vi "Initialize.vi"(8 "error in (no error)":errorcluster, 11 "Simple Actor in":refnum<class "Simple Actor.lvclass">) -> (0 "error out":errorcluster, 3 "Simple Actor out":refnum<class "Simple Actor.lvclass">)   [LabVIEW 2020, in "Simple Actor.lvlib" / "Simple Actor.lvclass"]
uses:
  Simple Actor.lvclass
  Execute Msg/Execute Msg.lvclass
  E:/NI I Program/Actor Intr Demo/Simple Actor/Actor Msg/Actor Msg.lvclass
  Simple Actor.lvclass/Simple Actor.ctl
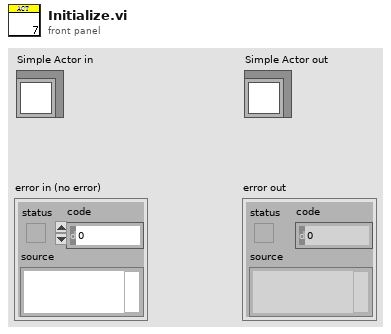
[diagram p1: front panel]
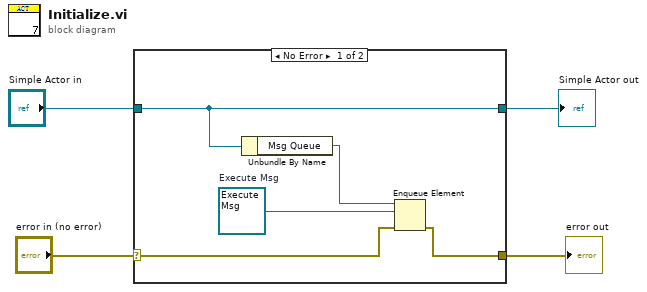
[diagram p0: block diagram]
diagram:
  n1 = case shown="No Error" "error in (no error)" {
    selector: "error in (no error)" -> [w6 w11]
    tunnel: [w5 w11] -> w3
    tunnel: [w9 w10] -> w1
    tunnel: "Simple Actor in" -> [w9 w10]
    frame No Error {
      w7 = refnum<class "Execute Msg.lvclass"> refnum  # Execute Msg
      n2 = Unbundle By Name(w9) -> ("Msg Queue"=w8:refnum<queue>)
      n3 = Enqueue Element(queue=w8, element=w7, error in (no error)=w6) -> (error out=w5:errorcluster)  [unwired: 1 in, 2 out]
    }
    frame Error {
    }
  }
  "error out" <- w3
  "Simple Actor out" <- w1
